vi "Digital_IO.vi"() -> ()   [LabVIEW 2018]
doc: "Discrete Controller Demo\nWritten for 2.14, Spring-2019"
uses:
  Components/TypeDefs/Select_TF.ctl
  Components/Controllers/TF_diff_mode.ctl
  <vilib>/Platform/TimedLoop/XDataNode/timing_clust.ctl
  <vilib>/Platform/TimedLoop/XDataNode/nitl_modes.ctl
  <vilib>/Platform/TimedLoop/XDataNode/wakeup.ctl
  <vilib>/myRIO/Instrument Drivers/Onboard IO/AO/typedefs/AO Reference.ctl
  <vilib>/myRIO/Common/Instrument Driver Framework/Utilities/typedefs/myRIO Generic Hardware Reference.ctl
  <vilib>/myRIO/Common/Instrument Driver Framework/Utilities/typedefs/Hardware Version Enum.ctl
  <vilib>/myRIO/Common/Instrument Driver Framework/Utilities/typedefs/myRIO v1.0 Reference.ctl
  <vilib>/myRIO/Common/Instrument Driver Framework/Utilities/typedefs/Generic FPGA Reference.ctl
  <vilib>/myRIO/Common/Instrument Driver Framework/myRIO v1.0/AO/typedefs/AO Channels List.ctl
  <vilib>/myRIO/Common/Instrument Driver Framework/myRIO v1.0/AO/typedefs/AO Channels Enum.ctl
  <vilib>/myRIO/Common/Instrument Driver Framework/Utilities/typedefs/Analog Scaling Constants List.ctl
  <vilib>/myRIO/Common/Instrument Driver Framework/Utilities/typedefs/Analog Scaling Constants.ctl
  <vilib>/userdefined/High Color/nirio_resource_hc.ctl
  <vilib>/myRIO/Instrument Drivers/Onboard IO/AI/typedefs/AI Reference.ctl
  <vilib>/myRIO/Common/Instrument Driver Framework/myRIO v1.0/AI/typedefs/AI Channels List.ctl
  <vilib>/myRIO/Common/Instrument Driver Framework/myRIO v1.0/AI/typedefs/AI Channels Enum.ctl
  <vilib>/myRIO/Common/Instrument Driver Framework/myRIO v1.0/AO/vis/myRIO v1.1 Open AO.vi
  <vilib>/myRIO/Common/Instrument Driver Framework/myRIO v1.0/AI/vis/myRIO v1.1 Open AI.vi
  <vilib>/myRIO/Common/Instrument Driver Framework/Utilities/vis/Validate Channels.vi
  <vilib>/myRIO/Common/Instrument Driver Framework/myRIO v1.0/AO/vis/myRIO v1.0 Reserve AO.vi
  <vilib>/myRIO/Common/Instrument Driver Framework/myRIO v1.0/AI/vis/myRIO v1.0 Reserve AI.vi
  <vilib>/myRIO/Common/Instrument Driver Framework/myRIO v1.0/AO/vis/myRIO v1.0 Close AO.vi
  <vilib>/myRIO/Common/Instrument Driver Framework/myRIO v1.0/AI/vis/myRIO v1.0 Close AI.vi
  <vilib>/myRIO/Common/Instrument Driver Framework/myRIO v1.0/AO/vis/myRIO v1.0 Build MUX Configuration AO.vi
  <vilib>/myRIO/Common/Instrument Driver Framework/myRIO v1.0/Resource Manager/vis/myRIO v1.0 Reserve Channel List.vi
  <vilib>/myRIO/Common/Instrument Driver Framework/myRIO v1.0/AI/vis/myRIO v1.0 Build MUX Configuration AI.vi
  <vilib>/myRIO/Common/Instrument Driver Framework/myRIO v1.0/AO/vis/myRIO v1.0 Unreserve AO.vi
  <vilib>/myRIO/Common/Instrument Driver Framework/myRIO v1.0/AI/vis/myRIO v1.0 Unreserve AI.vi
  <vilib>/myRIO/Common/Instrument Driver Framework/myRIO v1.0/Resource Manager/vis/myRIO v1.0 Reserve Channel.vi
  <vilib>/myRIO/Common/Instrument Driver Framework/myRIO v1.0/Resource Manager/vis/myRIO v1.0 Unreserve Channel.vi
  <vilib>/myRIO/Common/Instrument Driver Framework/myRIO v1.0/Resource Manager/vis/myRIO v1.0 Unreserve Channel List.vi
  <vilib>/myRIO/Common/Instrument Driver Framework/myRIO v1.0/Resource Manager/vis/myRIO v1.0 Build Mutex Name.vi
  <vilib>/Utility/VariantDataType/GetNumericInfo.vi
  <vilib>/Utility/error.llb/Error Cluster From Error Code.vi
  <vilib>/myRIO/Common/Instrument Driver Framework/myRIO v1.0/myRIO v1.1 Open.vi
  <vilib>/myRIO/Common/Instrument Driver Framework/myRIO v1.0/AI/vis/myRIO v1.0 Get Scaling Constants AI.vi
  <vilib>/myRIO/Common/Instrument Driver Framework/Utilities/vis/IO Manager.vi
  <vilib>/myRIO/Common/Instrument Driver Framework/Utilities/vis/Configuration Manager.vi
  <vilib>/myRIO/Common/Instrument Driver Framework/myRIO v1.0/myRIO v1.0 Close.vi
  <vilib>/myRIO/Common/Instrument Driver Framework/myRIO v1.0/AO/vis/myRIO v1.0 Get Scaling Constants AO.vi
  <vilib>/myRIO/Common/Instrument Driver Framework/myRIO v1.0/AI/vis/myRIO v1.0 Read AI.vi
  <vilib>/myRIO/Common/Instrument Driver Framework/myRIO v1.0/AO/vis/myRIO v1.0 Write AO.vi
  <vilib>/platform/TimedLoop/XDataNode/XDataNode.xnode
  <vilib>/myRIO/Instrument Drivers/Onboard IO/AI/vis/myRIO AI Open.xnode
  <vilib>/myRIO/Instrument Drivers/Onboard IO/AO/vis/myRIO AO Open.xnode
  <vilib>/Platform/TimedLoop/XDataNode/XDNodeRunTimeDep.lvlib
  <vilib>/myRIO/Instrument Drivers/Onboard IO/AI/AI.lvlib
  <vilib>/myRIO/Instrument Drivers/Onboard IO/AO/AO.lvlib
  components/Controllers/DiscreteControllers.lvlib
panel:
  in  "Mode":T1
  in  "Ti = 1/Ki [sec]":dbl=0.01
  out "Sample Time [s]":dbl format="%#_8f"
  out "# of loops late":i16
  in  "alpha":dbl=10.0
  in  "tau [sec]":dbl=0.001
  in  "Select discrete \ntransfer function":T2
  in  "System Stop Button":bool
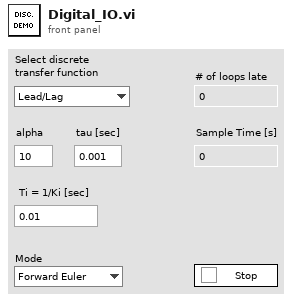
[diagram p1: front panel]
types:
  T1 = typedef "DiscreteControllers.lvlib/TF_diff_mode.ctl" = enum16{"Forward Euler", "Backward Euler", "Tustin (Bilinear)"}
  T2 = typedef "Select_TF.ctl" = enum16{"Lead/Lag", "Gain=20", "Unity", "Integrator"}
  T3 = typedef "XDNodeRunTimeDep.lvlib/timing_clust.ctl" = cluster{"Expected End [f-1]":u64, "Actual End [f-1]":u64, "Finished Late? [f-1]":bool, "Expected End [i-1]":u64, "Actual End [i-1]":u64, "Finished Late? [i-1]":bool, "Expected Start [i]":u64, "Actual Start [i]":u64, "Expected Start [f]":u64, "Actual Start [f]":u64, "Source Name":string, "Structure Name":string, "Period":i64, "Deadline":i64, "Offset":i64, "Start":i64, "Priority":i32, "Timeout":i32, "Mode":T4, "Wakeup Reason":T5, "Error":errorcluster, "Source Type":string, "Secondary Source Type":string, "Global End Time":u64, "Global Start Time":u64, "Frame Duration":u64, "Iteration Duration":u64, "Assigned CPU":i32, "I/O Scan Engine Mode":u32}
  T4 = typedef "XDNodeRunTimeDep.lvlib/nitl_modes.ctl" = enum32{"No Change", "Process missed periods, maintain original phase", "Discard missed periods, maintain original phase", "Process missed periods, ignore original phase", "Discard missed periods, ignore original phase"}
  T5 = typedef "XDNodeRunTimeDep.lvlib/wakeup.ctl" = enum32{"Normal", "Aborted", "Asynchronous wakeup", "Timing source error", "Timed loop error", "Timeout"}
  T6 = typedef "AI.lvlib/AI Reference.ctl" = cluster{"myRIO Reference":T7, "AI Channels List":T11, "AI Scaling Constants List":T13}
  T7 = typedef "myRIO Generic Hardware Reference.ctl" = cluster{"myRIO Model":T8, "myRIO Hardware Reference":T9}
  T8 = typedef "Hardware Version Enum.ctl" = enum16{"Unknown", "myRIO-1900", "myRIO-1950", "roboRIO", "NI ELVIS RIO CM", "ELVIS III"}
  T9 = typedef "myRIO v1.0 Reference.ctl" = cluster{"Generic FPGA Reference":T10, "Allow multiple opens":bool}
  T10 = typedef "Generic FPGA Reference.ctl" = refnum<k20>
  T11 = typedef "AI Channels List.ctl" = T12[]
  T12 = typedef "AI Channels Enum.ctl" = enum16{"Not Connected", "AudioIn/Left", "AudioIn/Right", "C/AI0", "C/AI1", "A/AI0", "A/AI1", "A/AI2", "A/AI3", "A/AI4", "A/AI5", "A/AI6", "A/AI7", "B/AI0", "B/AI1", "B/AI2", "B/AI3", "B/AI4", "B/AI5", "B/AI6", "B/AI7", "AI/AI0", "AI/AI1", "AI/AI2", "AI/AI3", "A/AI0 (DIFF)", "A/AI1 (DIFF)", "A/AI2 (DIFF)", "A/AI3 (DIFF)", "B/AI0 (DIFF)", "B/AI1 (DIFF)", "B/AI2 (DIFF)", "B/AI3 (DIFF)"}
  T13 = typedef "Analog Scaling Constants List.ctl" = T14[]
  T14 = typedef "Analog Scaling Constants.ctl" = cluster{"LSB Weight (Volts)":dbl, "Offset (Volts)":dbl, "Signed?":bool}
  T15 = typedef "AO.lvlib/AO Reference.ctl" = cluster{"myRIO Reference":T7, "AO Channel List":T16, "AO Scaling Constant List":T13}
  T16 = typedef "AO Channels List.ctl" = T17[]
  T17 = typedef "AO Channels Enum.ctl" = enum16{"Not Connected", "AudioOut/Left", "AudioOut/Right", "C/AO0", "C/AO1", "A/AO0", "A/AO1", "B/AO0", "B/AO1"}
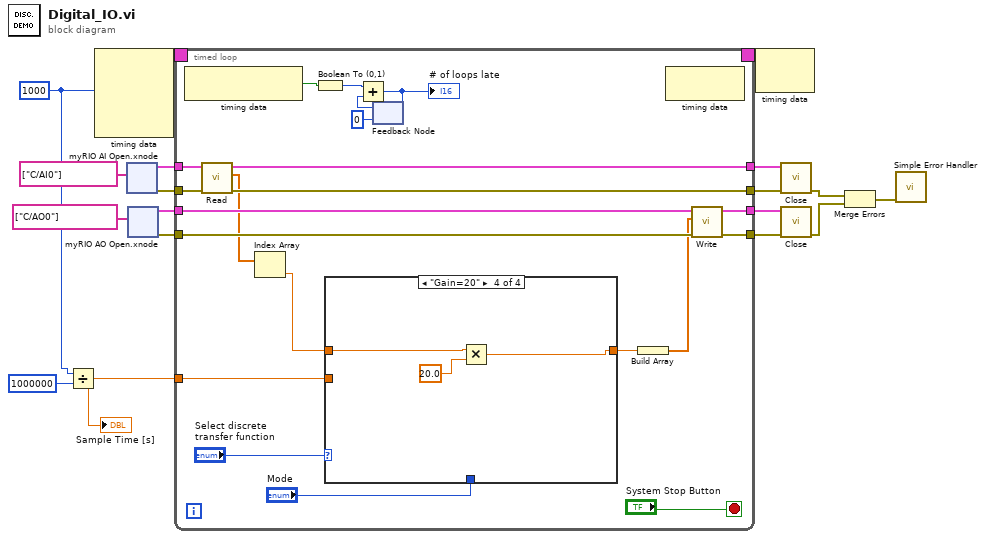
[diagram p0: block diagram]
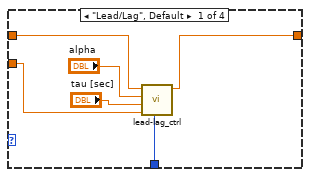
[diagram p2: hidden frame]
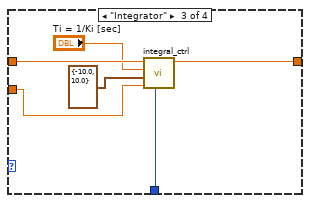
[diagram p4: hidden frame]
diagram:
  w2 = i64 1000 ("Period")
  n1 = Divide(x=w2, y=i64 1000000) -> (x/y=w1:dbl)
  "Sample Time [s]" <- w1
  n2 = node-c288(w2) -> (w18:T3)  [unwired: 3 in]
  n3 = xnode "myRIO AI Open.xnode"("Channel Names"=tag[] ["C/AI0"]) -> ("error out"=w14:errorcluster, "AI Ref Out"=w15:T6)  [unwired: 2 in]
  n4 = xnode "myRIO AO Open.xnode"("Channel Names"=tag[] ["C/AO0"]) -> ("error out"=w8:errorcluster, "AO Ref Out"=w10:T15)  [unwired: 2 in]
  n5 = timed-loop {
    timing: w18 -> [_]
    timing-out: [_] -> w17
    tunnel: w15 -> [w39]
    tunnel: w14 -> [w38]
    tunnel: [w37] -> w13
    tunnel: [w34] -> w12
    tunnel: w10 -> [w33]
    tunnel: [w32] -> w9
    tunnel: w8 -> [w31]
    tunnel: [w30] -> w7
    tunnel: w1 -> [w29]
    stop <- "System Stop Button" stop-if-true
    n6 = node-c288() -> (w24:bool)  [unwired: 1 in]
    n7 = call <vilib>:"Read.vi"("error in (no error)"=w38, "AI Ref In"=w39) -> ("error out"=w34:errorcluster, "Values"=w28:dbl[], "AI Ref Out"=w37:T6)  [unwired: 7 in]
    n8 = Index Array(array=w28) -> (element=w27:dbl)  [unwired: 1 in]
    n9 = Boolean To (0,1)(Boolean=w24) -> (0, 1=w23:i16)
    n10 = case shown="\"Gain=20\"" "Select discrete \ntransfer function" {
      tunnel: w29 -> [w42 _ w49 _]
      tunnel: w27 -> [w45 w46 w52 w55]
      tunnel: [w41 w46 w50 w54] -> w26
      tunnel: "Mode" -> [w40 _ w47 _]
      frame "Lead/Lag", Default {
        n11 = call "lead-lag_ctrl.vi"("Mode"=w40, "Sampling Time"=w42, "tau"="tau [sec]", "alpha"="alpha", "Input"=w45) -> ("Output"=w41:dbl)  [unwired: 5 in, 1 out]
      }
      frame "Unity" {
      }
      frame "Integrator" {
        n12 = call "integral_ctrl.vi"("Mode"=w47, "Sampling \nTime"=w49, "Anti-windup limits"=cluster{"Lower limit":dbl, "Upper limit":dbl} {"Lower limit"=-10.0, "Upper limit"=10.0}, "Ti"="Ti = 1/Ki [sec]", "Input"=w52) -> ("Output"=w50:dbl)  [unwired: 5 in, 1 out]
      }
      frame "Gain=20" {
        n13 = Multiply(x=w55, y=20.0) -> (x*y=w54:dbl)
      }
    }
    n14 = feedback #1(i16 0) -> (w21:i16)
    n15 = Add(x=w23, y=w21) -> (x+y=w22:i16)
    "# of loops late" <- w22
    n16 = feedback-in #1(w22) -> ()
    n17 = Build Array(w26) -> (w25:dbl[])
    n18 = node-c288() -> ()  [unwired: 1 in, 1 out]
    n19 = call <vilib>:"Write.vi"("error in (no error)"=w31, "Values"=w25, "AO Ref In"=w33) -> ("error out"=w30:errorcluster, "AO Ref Out"=w32:T15)  [unwired: 6 in]
  }
  n20 = node-c288(w17) -> ()  [unwired: 1 out]
  n21 = call <vilib>:"Close.vi"("error in (no error)"=w12, "AI Ref In"=w13) -> ("error out"=w5:errorcluster)  [unwired: 9 in]
  n22 = call <vilib>:"Close.vi"("error in (no error)"=w7, "AO Ref In"=w9) -> ("error out"=w4:errorcluster)  [unwired: 9 in]
  n23 = Merge Errors(w5, w4) -> (w3:errorcluster)
  n24 = call <vilib>:"Simple Error Handler.vi"("error in (no error)"=w3) -> ()  [unwired: 4 in, 5 out]
